vi "BWR_CMAP.vi"(9 "Brightness":dbl(slide) scale=0.0..255.0, 10 "Contrast":dbl(slide)=1.0 scale=0.0..255.0, 11 "Delta":dbl min=1.0 max=100.0) -> (3 "Cmap array":u32[](array[numeric]))   [LabVIEW 2018]
doc: "Connect \"Cmap array\" output to the intensity graph color table property node."
uses:
  <vilib>/Analysis/1siggen.llb/Ramp Pattern by Delta.vi
  <vilib>/Analysis/NI_AALBase.lvlib
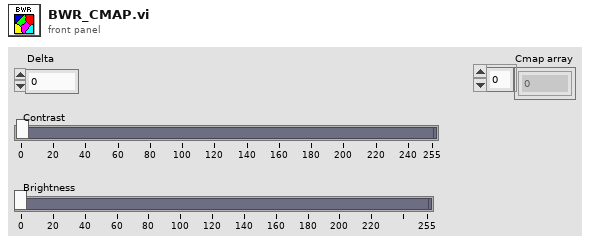
[diagram p1: front panel]
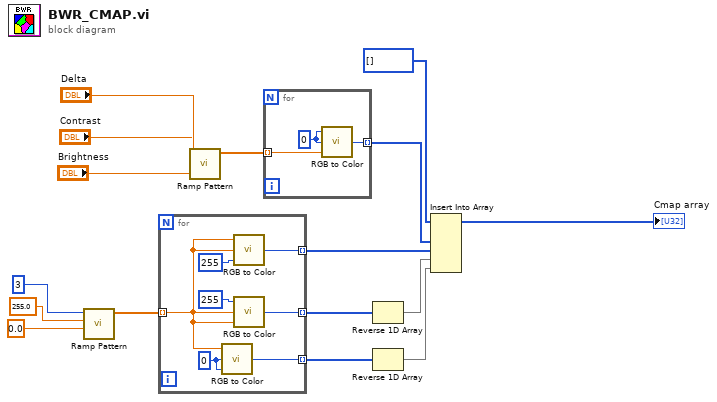
[diagram p0: block diagram]
diagram:
  n1 = call-poly <vilib>:"Ramp Pattern.vi"("start"=0.0, "end"=255.0, "delta"=3 ("samples")) -> ("Ramp Pattern"=w11:dbl[])  [unwired: 6 in, 2 out]
  n2 = for {
    tunnel: w11 -> [w18] mode=indexing
    tunnel: [w23] -> w5 mode=indexing
    tunnel: [w20] -> w10 mode=indexing
    tunnel: [w17] -> w12 mode=indexing
    w21 = u8 0 ("G")
    n3 = call <vilib>:"RGB to Color.vi"("B"=w21, "G"=w21, "R"=w18) -> ("Color"=w20:u32)
    n4 = call <vilib>:"RGB to Color.vi"("B"=u8 255, "G"=w18, "R"=w18) -> ("Color"=w17:u32)
    n5 = call <vilib>:"RGB to Color.vi"("B"=w18, "G"=w18, "R"=u8 255) -> ("Color"=w23:u32)
  }
  n6 = call-poly <vilib>:"Ramp Pattern.vi"("start"="Brightness", "end"="Contrast", "delta"="Delta") -> ("Ramp Pattern"=w1:dbl[])  [unwired: 6 in, 2 out]
  n7 = for {
    tunnel: w1 -> [w25] mode=indexing
    tunnel: [w26] -> w6 mode=indexing
    w24 = u8 0 ("R")
    n8 = call <vilib>:"RGB to Color.vi"("B"=w25, "G"=w24, "R"=w24) -> ("Color"=w26:u32)
  }
  n9 = Reverse 1D Array(array=w5) -> (reversed array=w7:u32[])
  n10 = Reverse 1D Array(array=w10) -> (reversed array=w8:u32[])
  n11 = Insert Into Array(array=u32[] [], new element #1=w6, new element #2=w12, new element #3=w7, new element #4=w8) -> (→"Cmap array":u32[])  [unwired: 1 in]
